vi "Open Connection.vi"(8 "error in":errorcluster, 11 "S7NetCom in":refnum<class "S7NetCom.lvclass">) -> (0 "error out":errorcluster, 3 "S7NetCom out":refnum<class "S7NetCom.lvclass">)   [LabVIEW 2014, in "S7NetCom.lvclass"]
doc: "Opens the network connection to the PLC, using the connection parameters passed to Create Object.vi.\n\n_____\nCopyright (c) 2019 Hampel Software Engineering (HSE), released under BSD license. More info can be found on https://dokuwiki.hampel-soft.com/code/hse/s7netcom. Original code published by Marc Christenson, Sisu Devices."
uses:
  S7NetCom.lvclass
  S7NetCom.lvclass/S7NetCom.ctl
  Controls/S7NetCom_ConnectionStatus.ctl
  Accessors/Set Connection Status.vi
  SubVIs/TPKT/TPKT - Write Packet.vi
  SubVIs/COTP/COTP - Read-Write Data.vi
  SubVIs/S7COMM/S7COMM - Add JOB Header to Params and Data.vi
  SubVIs/TPKT/TPKT - Add Header.vi
  Accessors/Get Timeout.vi
  Accessors/Get TCP Ref.vi
  Accessors/Set TCP Ref.vi
  SubVIs/COTP/COTP - Add Header.vi
  SubVIs/COTP/COTP - Validate Response Header.vi
  SubVIs/S7COMM/S7COMM - Create JOB Message Header.vi
  SubVIs/TPKT/TPKT - Header Bytes 1 and 2--constant.vi
  SubVIs/COTP/COTP - Header for Data Transfer--constant.vi
  SubVIs/COTP/COTP - Response Header Mismatch--error.vi
  SubVIs/S7COMM/S7COMM - Header - Protocol ID--constant.vi
  SubVIs/COTP/COTP - Build Connection Request Packet.vi
  SubVIs/TPKT/TPKT - Read Packet.vi
  SubVIs/S7COMM/S7COMM - Setup Communication Parameters--constant.vi
  SubVIs/S7COMM/S7COMM - Evaluate Setup Communication Response.vi
panel:
  # "More info on https://dokuwiki.hampel-soft.com/code/hse/s7netcom\n\nCopyright (c) 2019, HAMPEL SOFTWARE ENGINEERING (HSE)\nOriginal code developed by Marc Christenson, Sisu Devices\nAll rights reserved.\n\nRedistribution and use in source and binary forms, with or without\nmodification, are permitted provided that the following conditions are met:\n\n1. Redistributions of source code must retain the above copyright\n   notice, this list of conditions and the following disclaimer.\n\n2. Redistributions in binary form must reproduce the above copyright\n   notice, this list of conditions and the following disclaimer in the\n   documentation and/or other materials provided with the distribution.\n\n3. All advertising materials mentioning features or use of this software\n   must display the following acknowledgement:\n   This product includes software developed by HAMPEL SOFTWARE ENGINEERING.\n\n4. Neither the name of HAMPEL SOFTWARE ENGINEERING nor the\n   names of its contributors may be used to endorse or promote products\n   derived from this software without specific prior written permission.\n\nTHIS SOFTWARE IS PROVIDED BY HAMPEL SOFTWARE ENGINEERING ''AS IS'' AND ANY\nEXPRESS OR IMPLIED WARRANTIES, INCLUDING, BUT NOT LIMITED TO, THE IMPLIED\nWARRANTIES OF MERCHANTABILITY AND FITNESS FOR A PARTICULAR PURPOSE ARE\nDISCLAIMED. IN NO EVENT SHALL HAMPEL SOFTWARE ENGINEERING BE LIABLE FOR ANY\nDIRECT, INDIRECT, INCIDENTAL, SPECIAL, EXEMPLARY, OR CONSEQUENTIAL DAMAGES\n(INCLUDING, BUT NOT LIMITED TO, PROCUREMENT OF SUBSTITUTE GOODS OR SERVICES;\nLOSS OF USE, DATA, OR PROFITS; OR BUSINESS INTERRUPTION) HOWEVER CAUSED AND\nON ANY THEORY OF LIABILITY, WHETHER IN CONTRACT, STRICT LIABILITY, OR TORT\n(INCLUDING NEGLIGENCE OR OTHERWISE) ARISING IN ANY WAY OUT OF THE USE OF THIS\nSOFTWARE, EVEN IF ADVISED OF THE POSSIBILITY OF SUCH DAMAGE."
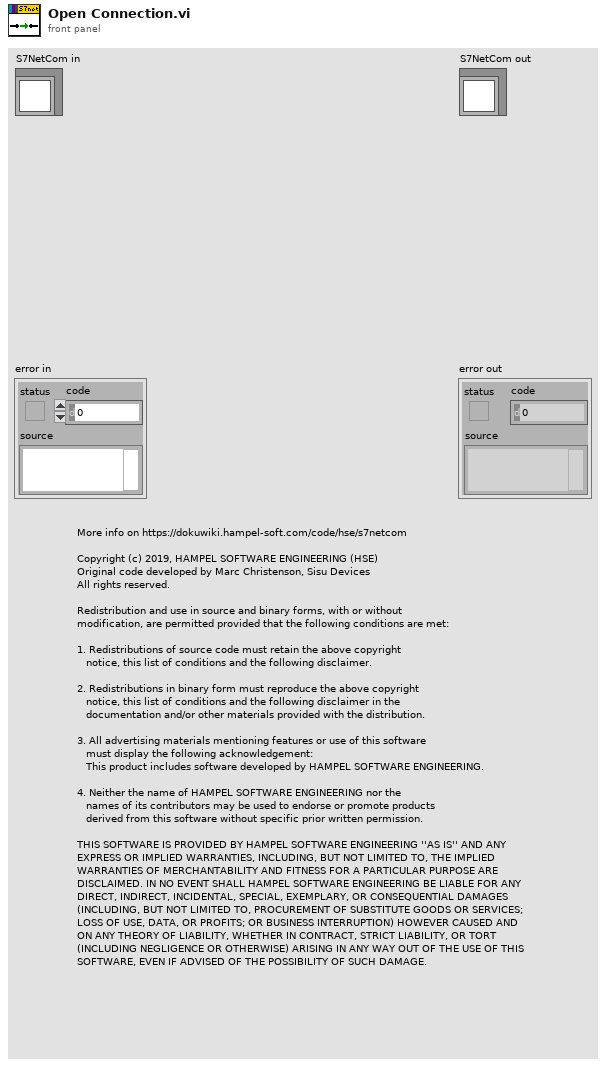
[diagram p1: front panel]
types:
  T1 = typedef "S7NetCom.lvclass/S7NetCom_ConnectionStatus.ctl" = enum16{"Connected", "Not Connected"}
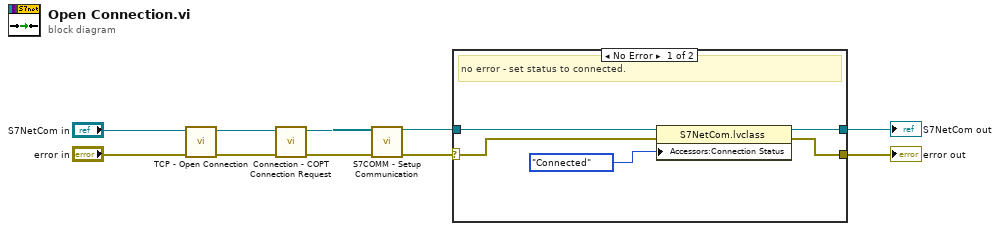
[diagram p0: block diagram]
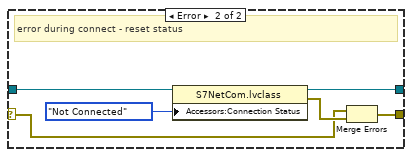
[diagram p2: hidden frame]
diagram:
  n1 = call "TCP - Open Connection.vi"("error in (no error)"="error in", "S7NetCom in"="S7NetCom in") -> ("error out"=w1:errorcluster, "S7NetCom out"=w2:refnum<class "S7NetCom.lvclass">)  [unwired: 8 in]
  n2 = call "Connection - COPT Connection Request.vi"("error in (no error)"=w1, "S7NetCom in"=w2) -> ("error out"=w3:errorcluster, "S7NetCom out"=w4:refnum<class "S7NetCom.lvclass">)  [unwired: 7 in, 1 out]
  n3 = call "S7COMM - Setup Communication.vi"("error in (no error)"=w3, "S7NetCom in"=w4) -> ("error out"=w10:errorcluster, "S7NetCom out"=w8:refnum<class "S7NetCom.lvclass">)  [unwired: 7 in, 1 out]
  n4 = case shown="No Error" w10 {
    selector: w10 -> [w15 w16]
    tunnel: w8 -> [w14 w21]
    tunnel: [w13 w20] -> w6
    tunnel: [w12 w17] -> w5
    frame No Error {
      # "no error - set status to connected."
      n5 = property class="S7NetCom.lvclass"(reference=w14, error in=w15, "Accessors:Connection Status"=S7NetCom_ConnectionStatus."Connected" ("Connection Status")) -> (reference out=w13:refnum<class "S7NetCom.lvclass">, error out=w12:errorcluster)
    }
    frame Error {
      # "error during connect - reset status"
      n6 = property class="S7NetCom.lvclass"(reference=w21, "Accessors:Connection Status"=S7NetCom_ConnectionStatus."Not Connected" ("Connection Status")) -> (reference out=w20:refnum<class "S7NetCom.lvclass">, error out=w19:errorcluster)  [unwired: 1 in]
      n7 = Merge Errors(w16, w19) -> (w17:errorcluster)
    }
  }
  "error out" <- w5
  "S7NetCom out" <- w6
